vi "uActor_Launch.vi"(6 "Show FP (F)":bool, 8 "error in (no error)":errorcluster, 10 "Actor to Launch":refnum<class "uActor.lvclass">, 11 "Caller Actor in":refnum<class "uActor.lvclass">) -> (0 "error out":errorcluster, 2 "uTransport_uActor":refnum<class "uTransport_uActor.lvclass">, 3 "Caller Actor out":refnum<class "uActor.lvclass">)   [LabVIEW 2023, in "uLib.lvlib" / "uActor.lvclass"]
doc: "Launch a new Actor. This will be a root actor if no caller actors are wired in."
uses:
  uActor.lvclass
  uTransport/uTransport_uActor/uTransport_uActor.lvclass
  uTransport/uTransport_uActor/uTransport_uActor.lvclass/uTransport_uActor.ctl
  uActor.lvclass/uActor.ctl
  uMsg/uMsg/uMsg.lvclass/uMsg.ctl
  uActor_SendMsg.vi
  uMsg/uMsg/uMsg Create.vi
  uTransport/uTransport_uActor/uTransport_uActor_SendMsg.vi
  uMsg/uMsg/uMsg Update Timestamp.vi
  uActor.vi
  uErr/uErr/uErr.lvclass
  uMsg/uMsg/uMsg.lvclass
  uData/uData/uData.lvclass
  uTransport/uTransport/uTransport.lvclass
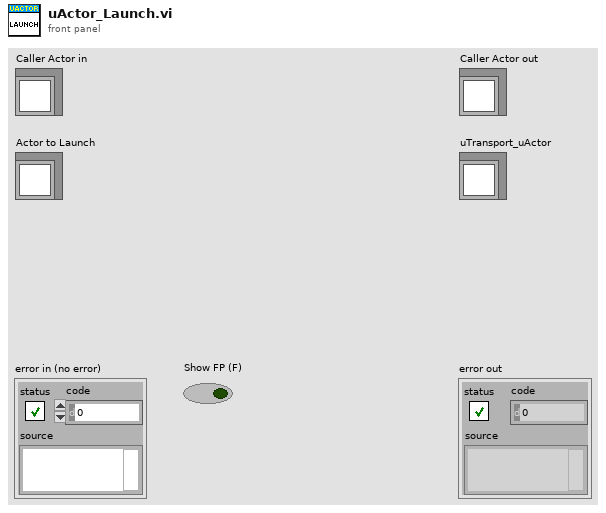
[diagram p1: front panel]
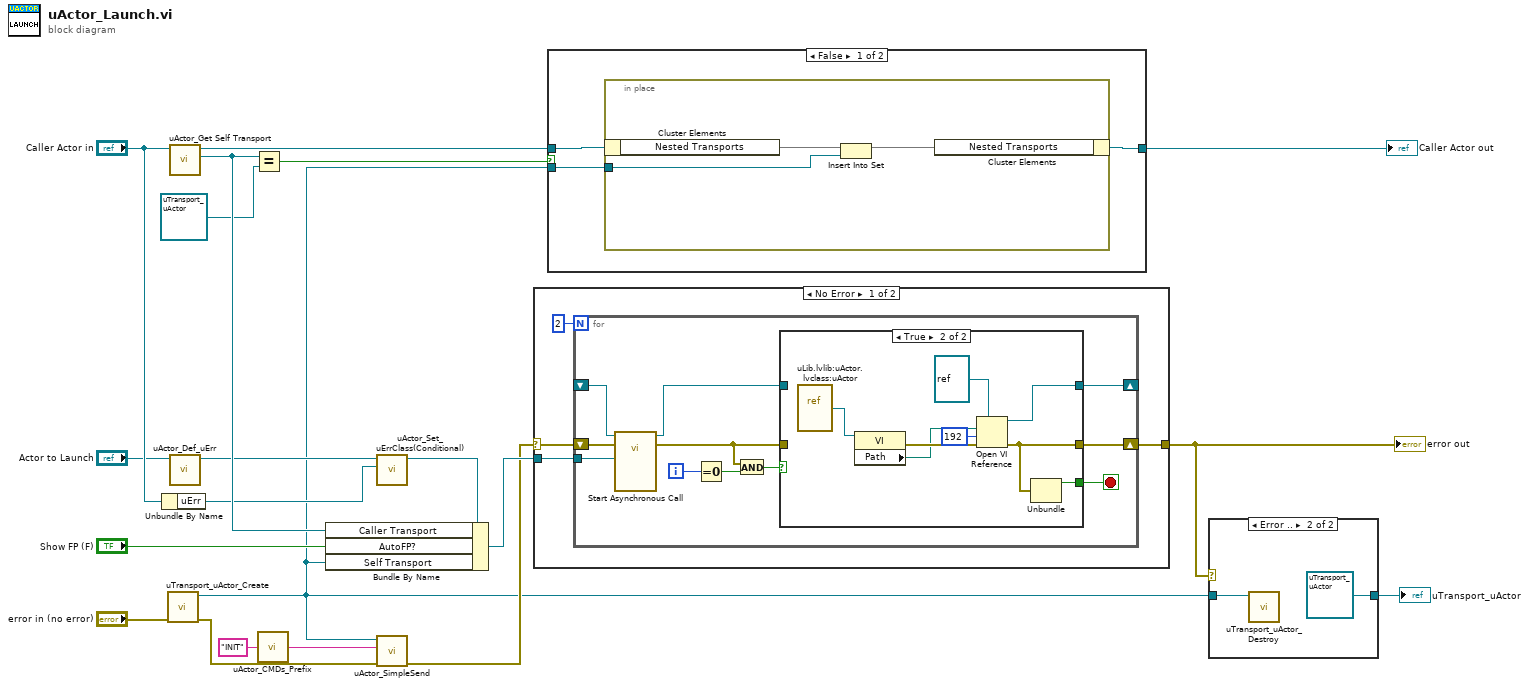
[diagram p0: block diagram]
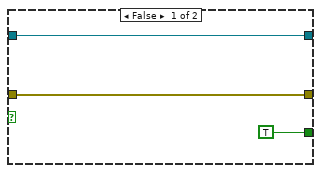
[diagram p2: hidden frame]
diagram:
  n1 = Unbundle By Name("Caller Actor in") -> ("uErr"=w5:refnum<class "uErr.lvclass">)
  n2 = call "uTransport_uActor_Create.vi"("error in (no error)"="error in (no error)") -> ("error out"=w20:errorcluster, "uTransport_uActor out"=w1:refnum<class "uTransport_uActor.lvclass">)  [unwired: 9 in]
  n3 = call "uActor_Get Self Transport.vi"("uActor in"="Caller Actor in") -> ("Actor Transport"=w16:refnum<class "uTransport_uActor.lvclass">, "uActor out"=w14:refnum<class "uActor.lvclass">)  [unwired: 9 in]
  n4 = call-dynamic "uActor_Def_uErr.vi"("uActor in"="Actor to Launch") -> ("uActor out"=w7:refnum<class "uActor.lvclass">)  [unwired: 9 in, 1 out]
  n5 = Equal?(x=w16, y=refnum<class "uTransport_uActor.lvclass"> refnum ("uFramework.lvlib:uTransport_uActor.lvclass")) -> (x = y?=w15:bool)
  n6 = call "uActor_CMDs_Prefix.vi"("uActor CMD"="INIT") -> ("Reserved CMD"=w3:string)
  n7 = call "uActor_Set_uErrClass(Conditional).vi"("uErr"=w5, "uActor in"=w7) -> ("uActor out"=w6:refnum<class "uActor.lvclass">)  [unwired: 9 in]
  n8 = Bundle By Name(cluster=w6, "Caller Transport"=w16, "AutoFP?"="Show FP (F)", "Self Transport"=w1) -> (w19:refnum<class "uActor.lvclass">)
  n9 = call "uActor_SimpleSend.vi"("error in (no error)"=w20, "Msg"=w3, "uActor Transport"=w1) -> ("error out"=w2:errorcluster)  [unwired: 8 in]
  n10 = case shown="No Error" w2 {
    selector: w2 -> [w21 w47]
    tunnel: w19 -> [w24 _]
    tunnel: [w23 w47] -> w12
    frame No Error {
      n11 = for {
        N: 2 -> [_]
        tunnel: w24 -> [w35]
        shift-right: [w31] -> w23
        shift-left: w21 -> [w34]
        shift-right: [w32] -> _
        shift-left: _ -> [w33]
        i -> [w30]
        stop <- w25 stop-if-true
        n12 = call-by-ref "Start Asynchronous Call"(reference=w33, error in=w34, "uActor in"=w35) -> (reference out=w29:refnum<vi>, error out=w26:errorcluster)  [unwired: 9 in, 2 out]
        n13 = Equal To 0?(x=w30) -> (x = 0?=w27:bool)
        n14 = And(x=w26, y=w27) -> (x .and. y?=w28:bool)
        n15 = case shown="True" w28 {
          tunnel: w26 -> [w37 _]
          tunnel: [w38 w41] -> w32
          tunnel: [w37 w40] -> w31
          tunnel: w29 -> [w38 _]
          tunnel: [TRUE w39] -> w25
          frame False {
          }
          frame True {
            n16 = vi-ref "uLib.lvlib:uActor.lvclass:uActor.vi"() -> (w43:refnum<vi>)
            n17 = property class="VI"(reference=w43) -> (error out=w46:errorcluster, "Path"=w45:path)  [unwired: 1 in, 1 out]
            n18 = Open VI Reference(type specifier VI Refnum (for type only)=refnum<vi> refnum, vi path=w45, options=192, error in (no error)=w46) -> (vi reference=w41:refnum<vi>, error out=w40:errorcluster)  [unwired: 2 in]
            n19 = Unbundle(w40) -> ("status"=w39:bool)  [unwired: 2 out]
          }
        }
      }
    }
    frame Error {
    }
  }
  "error out" <- w12
  n20 = case shown="False" w15 {
    tunnel: w14 -> [w50 w54]
    tunnel: [w48 w54] -> w13
    tunnel: w1 -> [w49 _]
    frame False {
      n21 = in-place {
        in-place-border: w49 -> [w51]
        n22 = in-place-cluster #1(w50) -> ("Nested Transports"=w52:set{refnum<class "uTransport_uActor.lvclass">})
        n23 = Insert Into Set(10:w51, 11:w52) -> (3:w53:set{refnum<class "uTransport_uActor.lvclass">})  [unwired: 1 out]
        n24 = in-place-cluster #1("Nested Transports"=w53) -> (w48:refnum<class "uActor.lvclass">)
      }
    }
    frame True {
      # "Attempting to launch a root actor. No caller provided."
    }
  }
  "Caller Actor out" <- w13
  n25 = case shown="Error .." w12 {
    tunnel: w1 -> [w55 w57]
    tunnel: [w55 refnum<class "uTransport_uActor.lvclass"> refnum] -> w18
    frame No Error {
    }
    frame Error {
      n26 = call "uTransport_uActor_Destroy.vi"("uTransport_uActor in"=w57) -> ()  [unwired: 9 in, 2 out]
    }
  }
  "uTransport_uActor" <- w18
